vi "Associate a File Extension.vi"(8 "error in (no error)":errorcluster, 10 "string":string=".myext", 11 "exe path":path) -> (0 "error out":errorcluster)   [LabVIEW 2014]
uses:
  <vilib>/registry/registry.llb/Registry RtKey.ctl
  <vilib>/registry/registry.llb/Write Registry Value Simple STR.vi
panel:
  out "concatenated string 2":string
  out "concatenated string":string
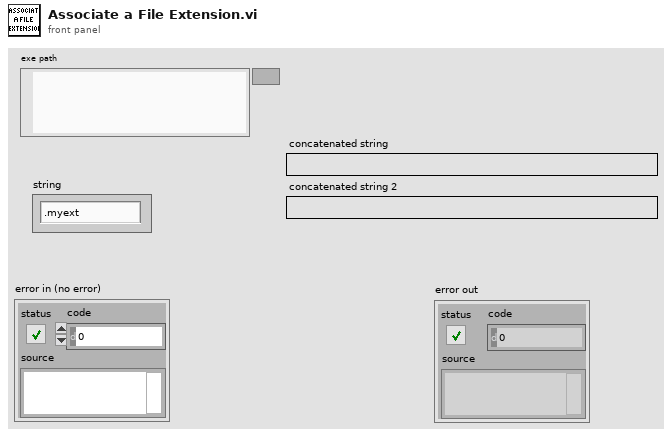
[diagram p1: front panel]
types:
  T1 = typedef "Registry RtKey.ctl" = enum32{"HKEY_CLASSES_ROOT", "HKEY_CURRENT_USER", "HKEY_LOCAL_MACHINE", "HKEY_USERS", "HKEY_PERFORMANCE_DATA", "HKEY_CURRENT_CONFIG", "HKEY_DYN_DATA"}
  T2 = typedef "Registry refnum.ctl" = refnum<k1>
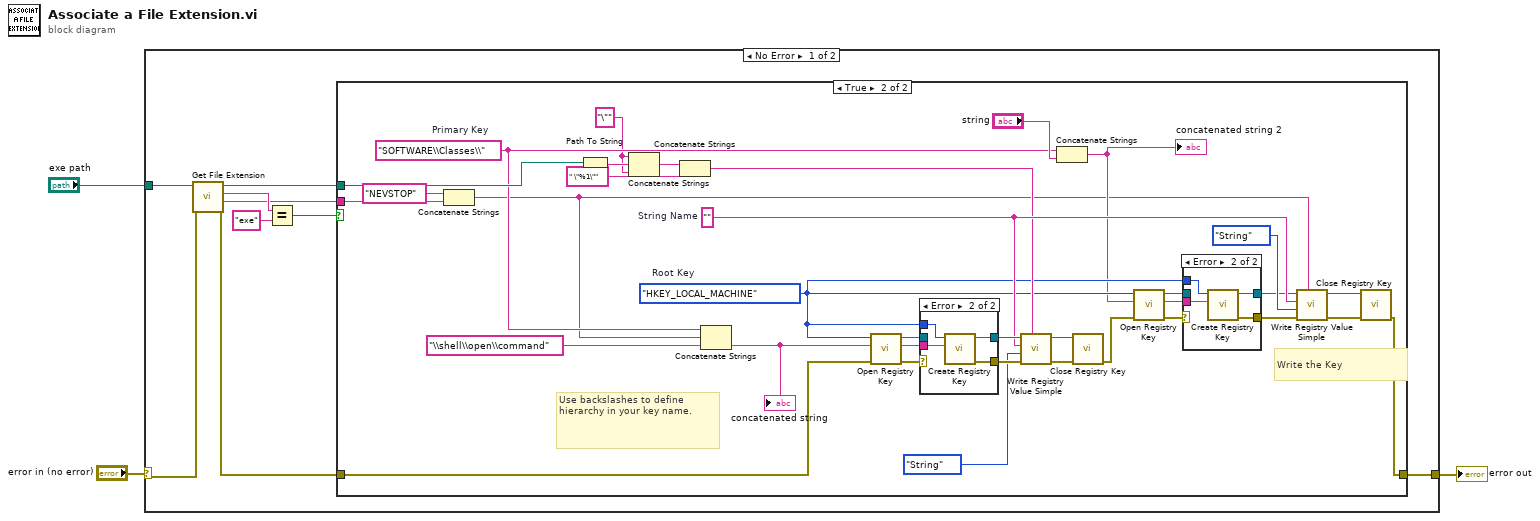
[diagram p0: block diagram]
diagram:
  n1 = case shown="No Error" "error in (no error)" {
    selector: "error in (no error)" -> [w8 w59]
    tunnel: [w12 w59] -> w3
    tunnel: "exe path" -> [w11 _]
    frame No Error {
      n2 = call <vilib>:"Get File Extension.vi"("error in (no error)"=w8, "file"=w11) -> ("error out"=w7:errorcluster, "filename without extension"=w4:string, "lowercase file extension"=w5:string, "dup file"=w6:path)  [unwired: 6 in]
      n3 = Equal?(x=w5, y="exe") -> (x = y?=w9:bool)
      n4 = case shown="True" w9 {
        tunnel: [w13 w37] -> w12
        tunnel: w7 -> [w13 w29]
        tunnel: w4 -> [_ w20]
        tunnel: w6 -> [_ w35]
        frame False {
        }
        frame True {
          w14 = "\"" ("string")
          w18 = "SOFTWARE\\Classes\\"  # Primary Key
          w36 = ""  # String Name
          w22 = Registry_RtKey."HKEY_LOCAL_MACHINE"  # Root Key
          # "Use backslashes to define hierarchy in your key name."
          # "Write the Key"
          n5 = Concatenate Strings("NEVSTOP" ("string"), w20) -> (w17:string)
          n6 = Path To String(path=w35) -> (string=w34:string)
          n7 = Concatenate Strings(w14, w34, w14) -> (w15:string)
          n8 = Concatenate Strings(w15, " \"%1\"" ("string")) -> (w32:string)
          n9 = Concatenate Strings(w18, w17, "\\shell\\open\\command" ("subkey")) -> (w30:string)
          "concatenated string" <- w30
          n10 = call <vilib>:"Open Registry Key.vi"("error in (no error)"=w29, "subkey"=w30, "root key (HKEY_LOCAL_MACHINE)"=w22) -> ("error out"=w28:errorcluster, "refnum out"=w27:T2)  [unwired: 7 in]
          n11 = case shown="Error" w28 {
            selector: w28 -> [w54 _]
            tunnel: [w54 w58] -> w45
            tunnel: [w53 w57] -> w43
            tunnel: w22 -> [_ w56]
            tunnel: w30 -> [_ w55]
            tunnel: w27 -> [w53 _]
            frame No Error {
            }
            frame Error {
              n12 = call <vilib>:"Create Registry Key.vi"("subkey"=w55, "root key (HKEY_LOCAL_MACHINE)"=w56) -> ("error out"=w58:errorcluster, "refnum out"=w57:T2)  [unwired: 7 in, 1 out]
            }
          }
          n13 = call-poly <vilib>:"Write Registry Value Simple.vi"("String/Binary data"=w32, "error in (no error)"=w45, "simple data type"=enum16{"String", "Binary", "DWORD"}."String", "value"=w36, "refnum"=w43) -> ("error out"=w41:errorcluster, "refnum out"=w42:T2)  [unwired: 3 in]
          n14 = Concatenate Strings(w18, "string") -> (w19:string)
          "concatenated string 2" <- w19
          n15 = call <vilib>:"Close Registry Key.vi"("error in (no error)"=w41, "refnum"=w42) -> ("error out"=w21:errorcluster)  [unwired: 5 in]
          n16 = call <vilib>:"Open Registry Key.vi"("error in (no error)"=w21, "subkey"=w19, "root key (HKEY_LOCAL_MACHINE)"=w22) -> ("error out"=w25:errorcluster, "refnum out"=w26:T2)  [unwired: 7 in]
          n17 = case shown="Error" w25 {
            selector: w25 -> [w48 _]
            tunnel: [w48 w52] -> w24
            tunnel: [w47 w51] -> w23
            tunnel: w22 -> [_ w50]
            tunnel: w19 -> [_ w49]
            tunnel: w26 -> [w47 _]
            frame No Error {
            }
            frame Error {
              n18 = call <vilib>:"Create Registry Key.vi"("subkey"=w49, "root key (HKEY_LOCAL_MACHINE)"=w50) -> ("error out"=w52:errorcluster, "refnum out"=w51:T2)  [unwired: 7 in, 1 out]
            }
          }
          n19 = call-poly <vilib>:"Write Registry Value Simple.vi"("String/Binary data"=w17, "error in (no error)"=w24, "simple data type"=enum16{"String", "Binary", "DWORD"}."String", "value"=w36, "refnum"=w23) -> ("error out"=w40:errorcluster, "refnum out"=w39:T2)  [unwired: 3 in]
          n20 = call <vilib>:"Close Registry Key.vi"("error in (no error)"=w40, "refnum"=w39) -> ("error out"=w37:errorcluster)  [unwired: 5 in]
        }
      }
    }
    frame Error {
    }
  }
  "error out" <- w3
